vi "User Log In (popup).vi"(8 "error in (no error)":errorcluster, 11 "?":path) -> (0 "error out":errorcluster, 3 "User-data cluster Out":T1)   [LabVIEW 2012]
uses:
  SubVIs/typedef/User Accounts.ctl
  SubVIs/typedef/User_Data_Cluster.ctl
panel:
  in  "wrong user":string
  in  "wrong pass":string
  in  "maxx attemps":string
  in  "User-data cluster":T1
  in  "?":bool
  in  "?":bool
  in  "Password":string
  in  "Usuario":string
  in  "Cluster 3":T3
  out "Attempt (Max)":dbl
  out "Attempt":dbl
  # "Log In attempt"
  # "of"
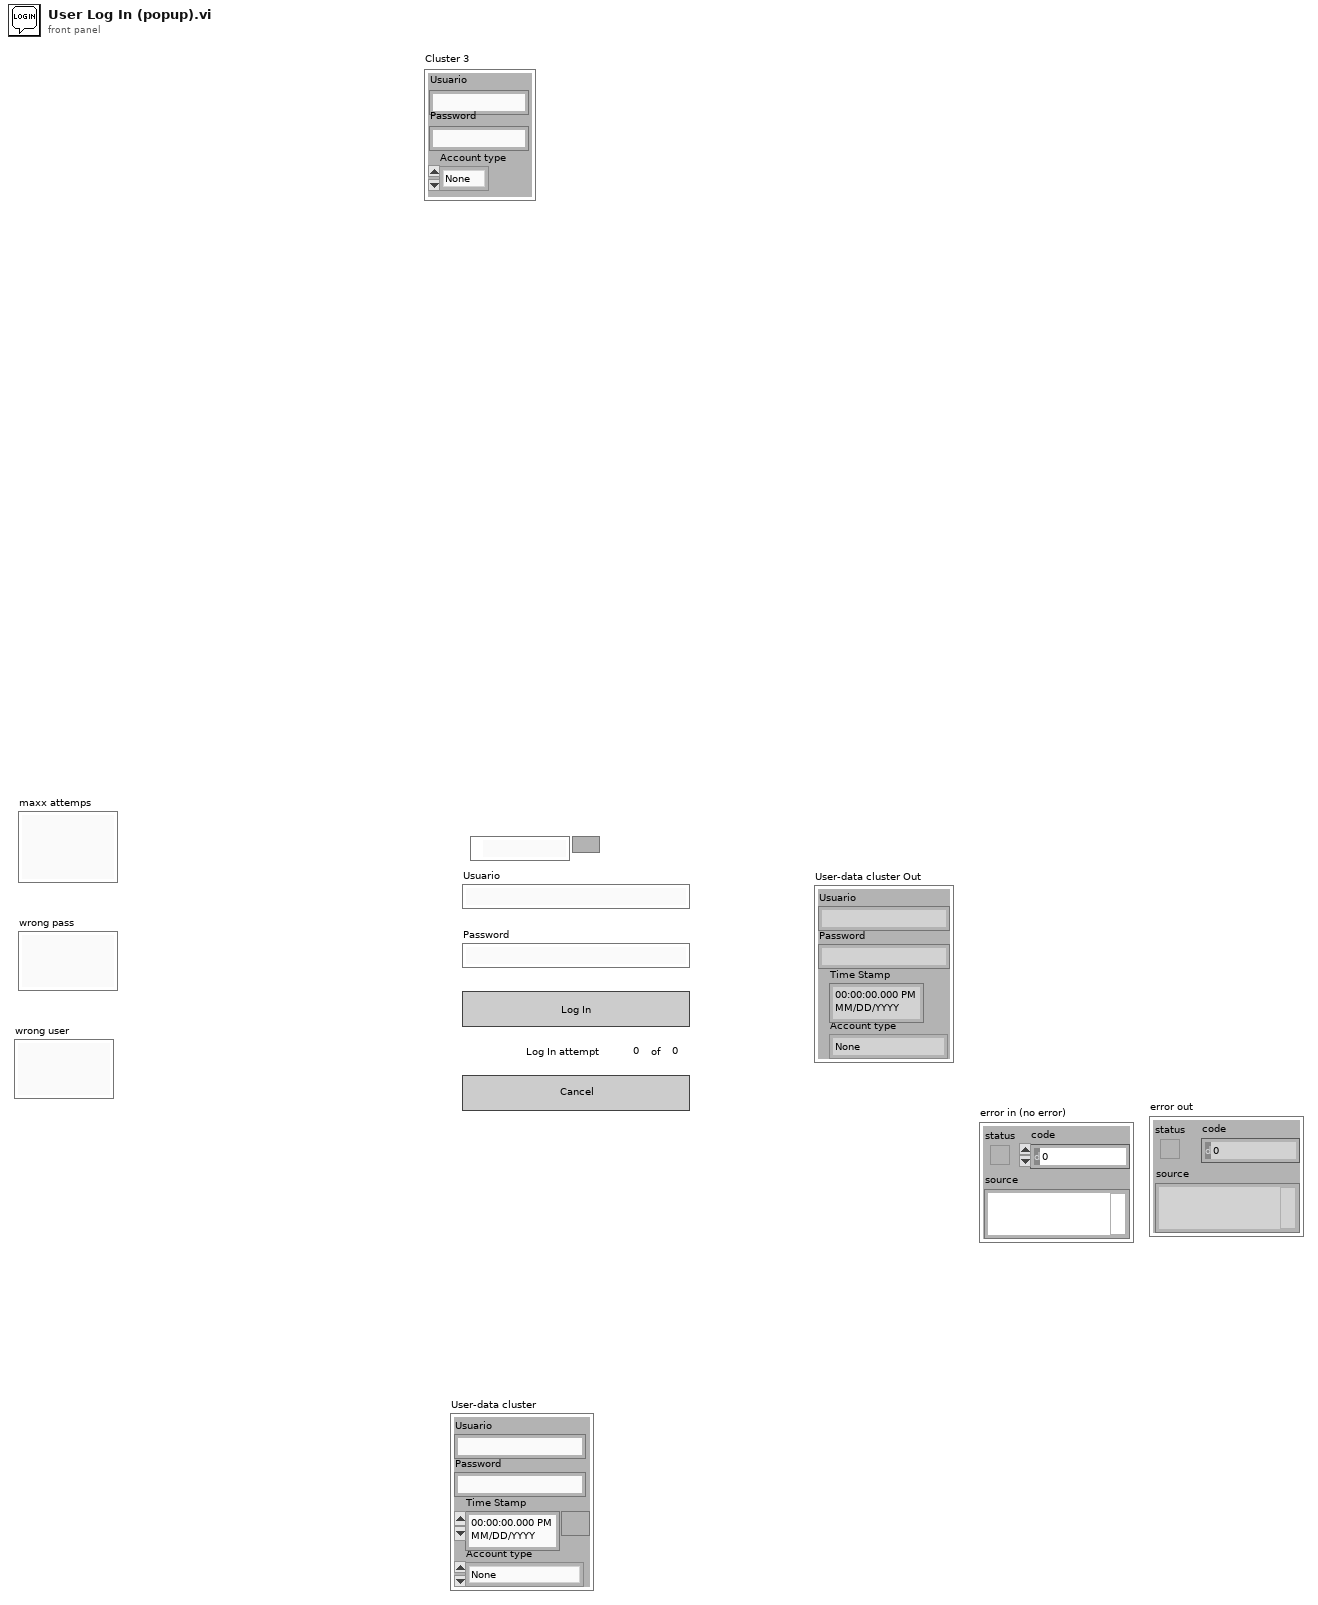
[diagram p1: front panel]
types:
  T1 = typedef "User_Data_Cluster.ctl" = cluster{"Usuario":string, "Password":string, "Account type":T2, "Time Stamp":timestamp}
  T2 = typedef "User Accounts.ctl" = enum16{"None", "User", "Admin"}
  T3 = cluster{"Usuario":string, "Password":string, "Account type":T2}
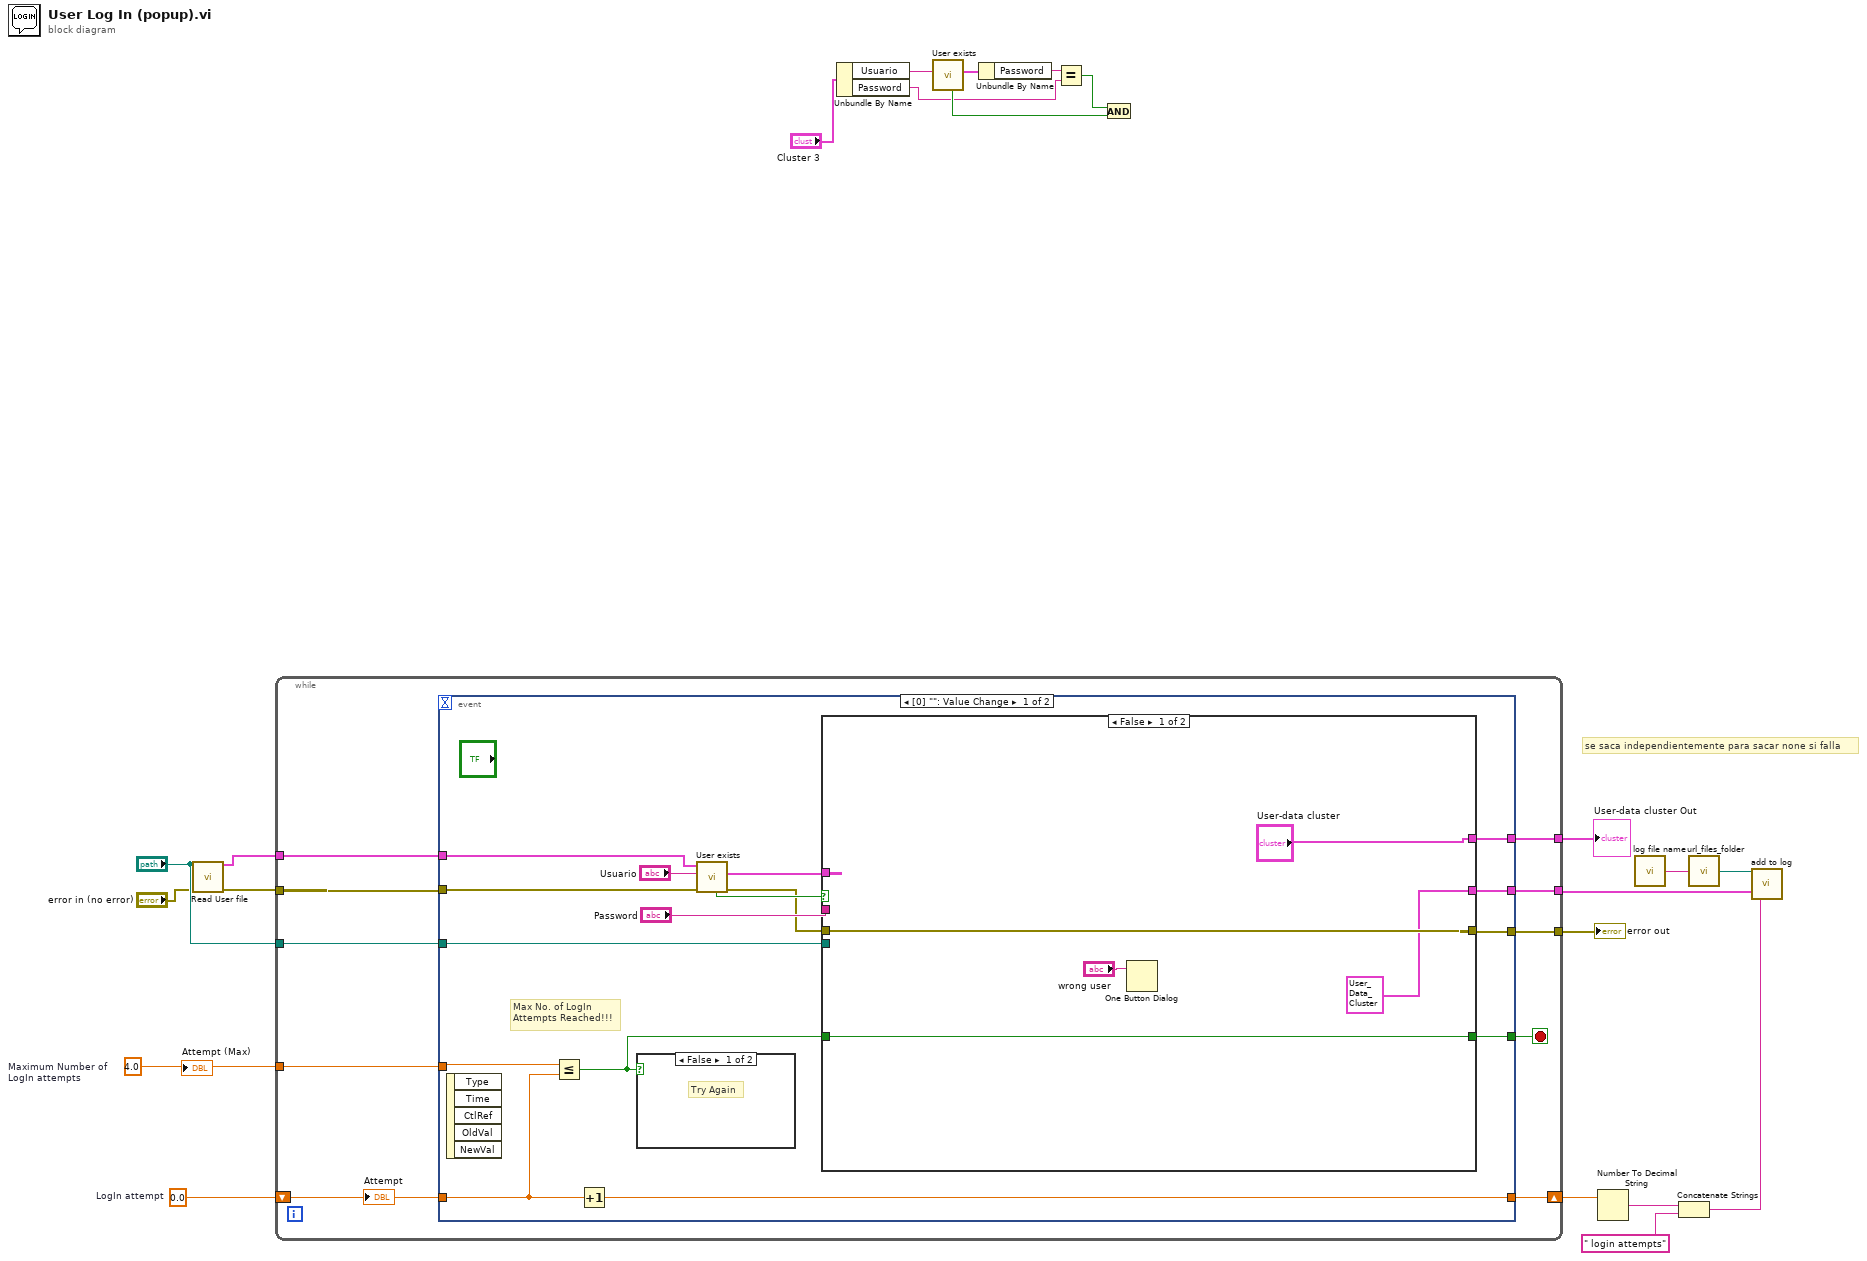
[diagram p0: block diagram]
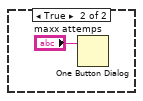
[diagram p2: hidden frame]
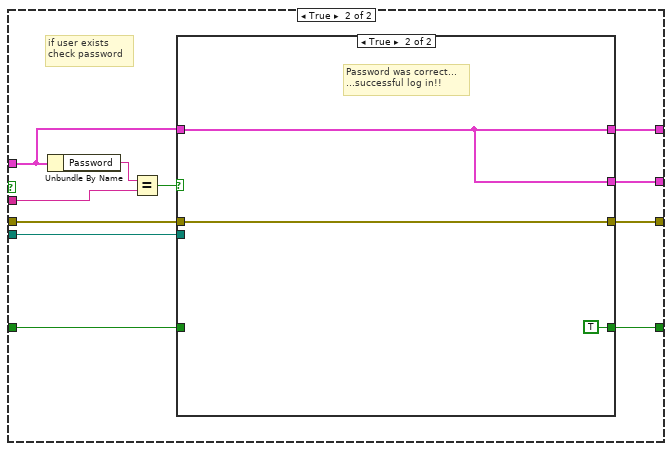
[diagram p3: hidden frame]
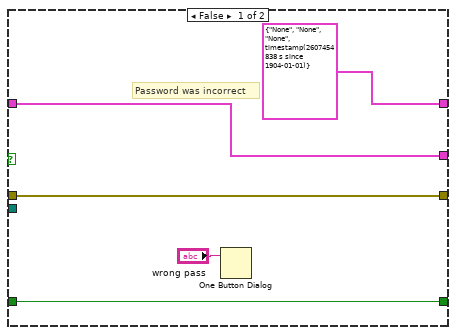
[diagram p4: hidden frame]
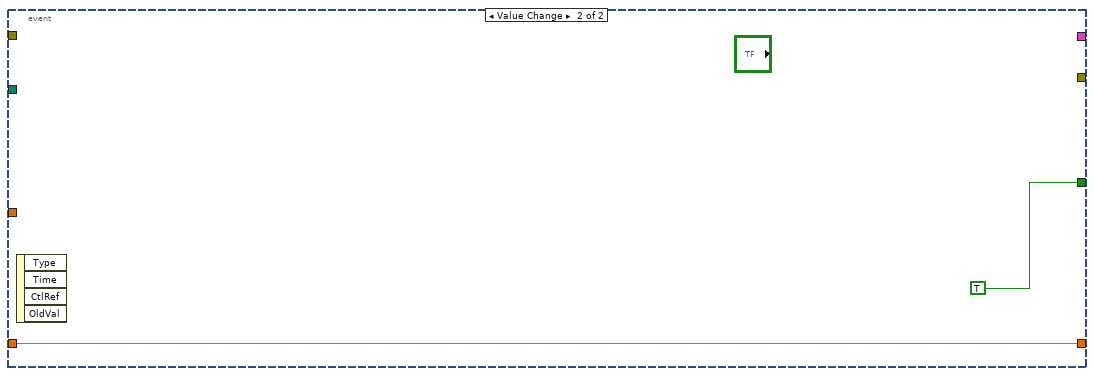
[diagram p5: hidden frame]
diagram:
  w22 = 0.0  # LogIn attempt
  w7 = 4.0  # Maximum Number of  LogIn attempts
  # "se saca independientemente para sacar none si falla"
  n1 = call "Read User file.vi"("file path (use dialog)"="?", "error in"="error in (no error)") -> ("Array"=w5:T1[], "error out"=w8:errorcluster)  [unwired: 12 in]
  n2 = while {
    tunnel: w7 -> [w29]
    shift-right: [w31] -> w6
    shift-left: w22 -> [w32]
    tunnel: w8 -> [w26]
    tunnel: [w25] -> w21
    tunnel: w5 -> [w28]
    tunnel: "?" -> [w27]
    tunnel: [w24] -> w12
    tunnel: [w23] -> w1
    stop <- w30 stop-if-true
    n3 = event shown="[0] \"\": Value Change" {
      selector: _ -> [_ _]
      dyn-events: _ -> [_ _]
      timeout: _ -> [_ _]
      tunnel: w32 -> [w35 w75]
      tunnel: [w37 w75] -> w31
      tunnel: [w48 TRUE] -> w30
      tunnel: w29 -> [w36 _]
      tunnel: w28 -> [w43 _]
      tunnel: w27 -> [w42 _]
      tunnel: w26 -> [w41 _]
      tunnel: [w40 _] -> w25
      tunnel: [w38 _] -> w24
      tunnel: [w34 _] -> w23
      event Value Change {
        # "Max No. of LogIn\nAttempts Reached!!!"
        n4 = event-data() -> ()  [unwired: 1 in, 5 out]
        n5 = Less Or Equal?(x=w36, y=w35) -> (x <= y?=w33:bool)
        n6 = Increment(x=w35) -> (x+1=w37:dbl)
        n7 = case shown="False" w33 {
          frame False {
            # "Try Again"
          }
          frame True {
            n8 = One Button Dialog(message="maxx attemps") -> ()  [unwired: 1 in, 1 out]
          }
        }
        n9 = call "User exists.vi"("error in"=w41, "user"="Usuario", "Array"=w43) -> ("error out"=w39:errorcluster, "User-data cluster"=w45:T1, "exist?"=w44:bool)  [unwired: 5 in, 1 out]
        n10 = case shown="False" w44 {
          tunnel: [w51 w65] -> w48
          tunnel: "Password" -> [_ w64]
          tunnel: w45 -> [_ w61]
          tunnel: w42 -> [_ w60]
          tunnel: [w54 w59] -> w40
          tunnel: w39 -> [w54 w58]
          tunnel: [T1 {"Usuario"="", "Password"="", "Account type"=enum."None", "Time Stamp"=timestamp(2607442386.535288 s since 1904-01-01)} ("element") w57] -> w38
          tunnel: w33 -> [w51 w56]
          tunnel: ["User-data cluster" w55] -> w34
          frame False {
            n11 = One Button Dialog(message="wrong user") -> ()  [unwired: 1 in, 1 out]
          }
          frame True {
            # "if user exists\ncheck password"
            n12 = Unbundle By Name(w61) -> ("Password"=w63:string)
            n13 = Equal?(x=w63, y=w64) -> (x = y?=w62:bool)
            n14 = case shown="True" w62 {
              tunnel: [w67 TRUE] -> w65
              tunnel: w61 -> [w68 w73]
              tunnel: w60 -> [_ _]
              tunnel: [w70 w72] -> w59
              tunnel: w58 -> [w70 w72]
              tunnel: [w68 w73] -> w57
              tunnel: w56 -> [w67 _]
              tunnel: [T1 {"Usuario"="None", "Password"="None", "Account type"=enum."None", "Time Stamp"=timestamp(2607454838.413 s since 1904-01-01)} ("User-data cluster") w73] -> w55
              frame False {
                # "Password was incorrect"
                n15 = One Button Dialog(message="wrong pass") -> ()  [unwired: 1 in, 1 out]
              }
              frame True {
                # "Password was correct...\n...successful log in!!"
              }
            }
          }
        }
      }
      event Value Change {
        n16 = event-data() -> ()  [unwired: 1 in, 4 out]
      }
    }
    "Attempt" <- w32
  }
  "error out" <- w21
  "User-data cluster Out" <- w1
  n17 = Unbundle By Name("Cluster 3") -> ("Usuario"=w19:string, "Password"=w14:string)
  n18 = call "User exists.vi"("user"=w19) -> ("User-data cluster"=w18:T1, "exist?"=w16:bool)  [unwired: 7 in, 2 out]
  n19 = Unbundle By Name(w18) -> ("Password"=w17:string)
  n20 = Equal?(x=w17, y=w14) -> (x = y?=w15:bool)
  n21 = And(x=w15, y=w16) -> ()  [unwired: 1 out]
  n22 = Number To Decimal String(number=w6) -> (decimal integer string=w3:string)  [unwired: 1 in]
  n23 = call "log file name.vi"() -> ("file name"=w10:string)  [unwired: 15 in]
  n24 = Concatenate Strings(w3, " login attempts" ("string")) -> (w4:string)
  n25 = call "url_files_folder.vi"("file name"=w10) -> ("Path"=w11:path)  [unwired: 14 in]
  n26 = call "add to log.vi"("Path"=w11, "User-data cluster"=w12, "Data"=w4) -> ()  [unwired: 13 in]
  "Attempt (Max)" <- w7
